vi "בדיקת מתח תפיסה של סליל פיקוד ללא עומס 5.vi"(8 "error":errorcluster, 10 "lines":tag="PXI1Slot8/port0/line1", 11 "Path for Log":path) -> (0 "error out":errorcluster, 1 "מצב ממסר פתוח/סגור":bool, 2 "מתח סגירת הממסר":dbl format="%.4f", 3 "מתח מוצא מהספק":dbl format="%.4f", 5 "resultUserPrompt":bool)   [LabVIEW 2015]
uses:
  <vilib>/DAQmx/write.llb/DAQmx Write (Digital Bool 1Line 1Point).vi
  <vilib>/DAQmx/create/channels.llb/DAQmx Create Channel (DO-Digital Output).vi
  <vilib>/DAQmx/miscellaneous.llb/DAQmx Fill In Error Info.vi
panel:
  out "progress":dbl(slide) scale=0.0..36.0
  out "error IO DMM":errorcluster
  in  "Stop Button":bool
  # "Right-Click to\nexplain error"
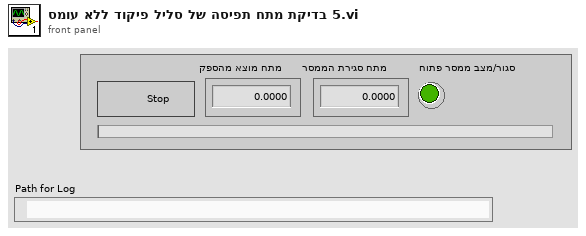
[diagram p1: front panel]
types:
  T1 = enum32{"Invalid", "Standard", "Closed", "Hidden", "Minimized", "Maximized"}
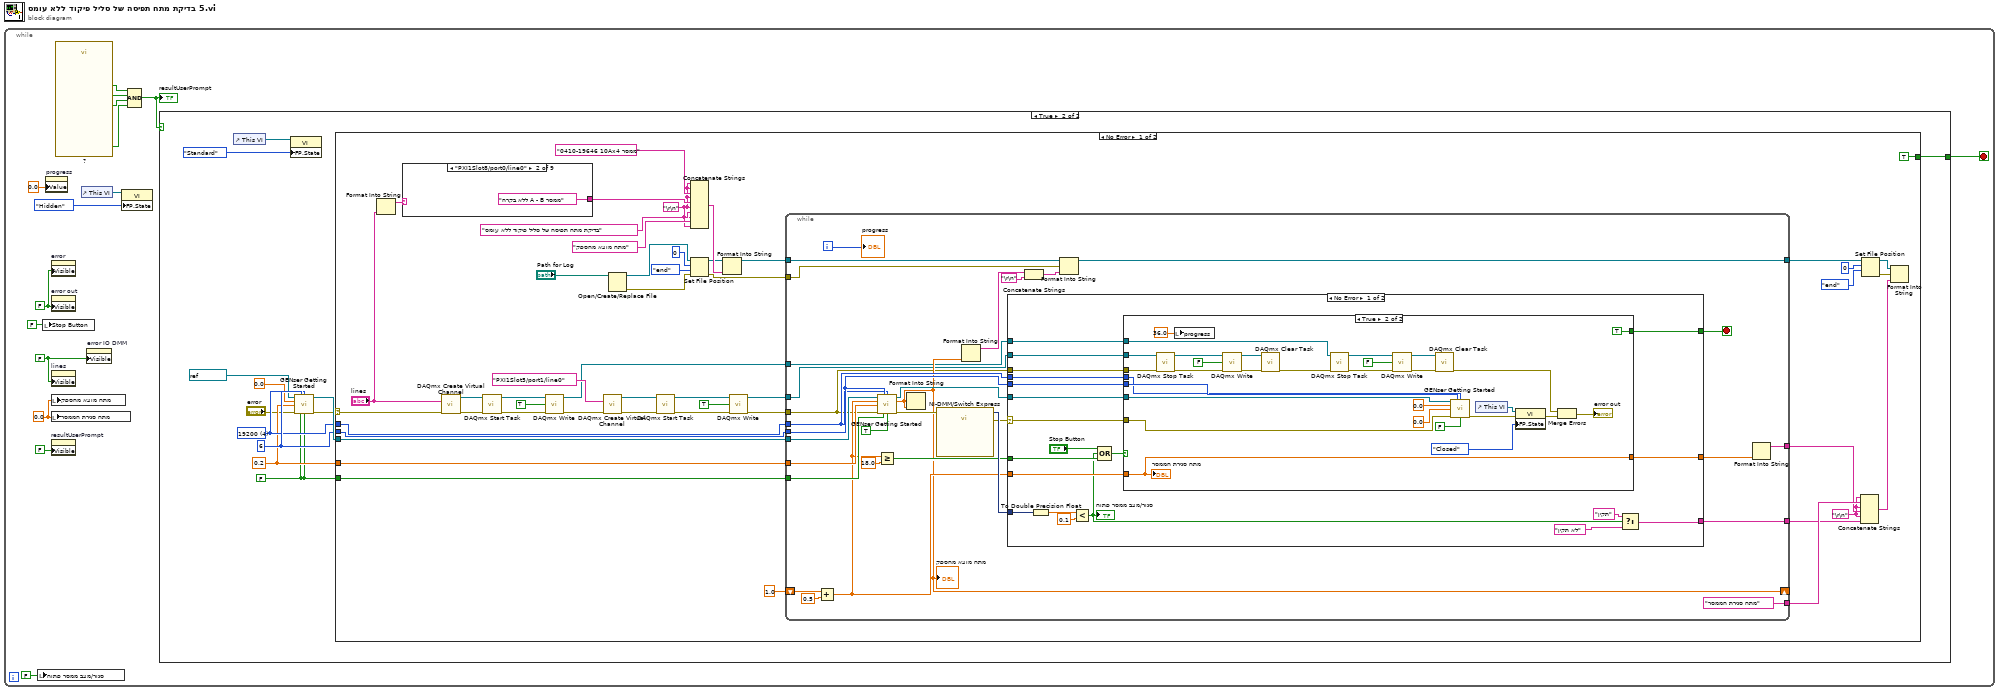
[diagram p0: block diagram]
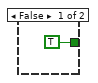
[diagram p2: hidden frame]
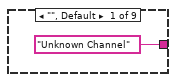
[diagram p3: hidden frame]
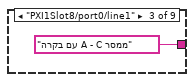
[diagram p4: hidden frame]
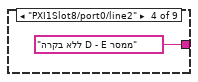
[diagram p5: hidden frame]
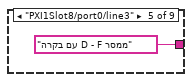
[diagram p6: hidden frame]
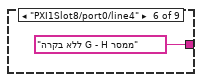
[diagram p7: hidden frame]
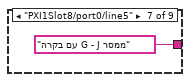
[diagram p8: hidden frame]
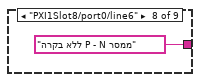
[diagram p9: hidden frame]
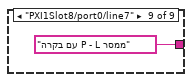
[diagram p10: hidden frame]
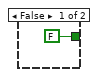
[diagram p11: hidden frame]
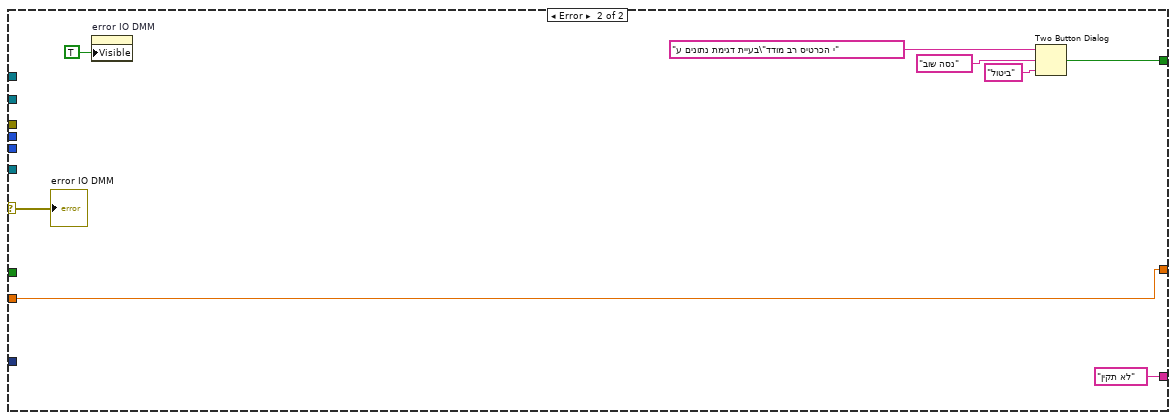
[diagram p12: hidden frame]
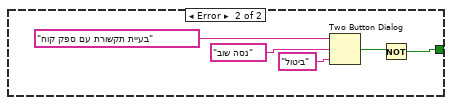
[diagram p13: hidden frame]
diagram:
  n1 = while {
    stop <- w1 stop-if-true
    w4 = FALSE ("Visible")
    w9 = 0.0 ("signals out")
    w2 = FALSE ("Visible")
    n2 = local write "מצב ממסר פתוח/סגור"(FALSE ("מגע סגור")) -> ()
    n3 = local write "Stop Button"(FALSE ("Reset (T)")) -> ()
    n4 = property on="progress" class="Slide (strict)"("Value"=0.0 ("progress")) -> ()  [unwired: 2 in, 2 out]
    n5 = property on="error" class="Clust (strict)"("Visible"=w4) -> ()  [unwired: 2 in, 2 out]
    n6 = property on="error out" class="Clust (strict)"("Visible"=w4) -> ()  [unwired: 2 in, 2 out]
    n7 = property on="lines" class="DAQmxName"("Visible"=w2) -> ()  [unwired: 2 in, 2 out]
    n8 = local write "מתח מוצא מהספק"(w9) -> ()
    n9 = local write "מתח סגירת הממסר"(w9) -> ()
    n10 = property on="resultUserPrompt" class="Bool (strict)"("Visible"=FALSE) -> ()  [unwired: 2 in, 2 out]
    n11 = call "?"() -> ("הדקי הרב מודד"=w7:bool, "M מגע שלילי"=w13:bool, "K מגע חיובי"=w14:bool, "OK"=w8:bool)  [unwired: 15 in, 1 out]
    n12 = control-ref of="This VI"() -> (w6:refnum<vi>)
    n13 = property on="error IO DMM" class="Clust (strict)"("Visible"=w2) -> ()  [unwired: 2 in, 2 out]
    n14 = property class="VI"(reference=w6, "FP.State"=T1."Hidden" ("Front Panel Window:State")) -> ()  [unwired: 1 in, 2 out]
    n15 = Compound Arithmetic op=AND(w8, w14, w13, w7) -> (w15:bool)
    "resultUserPrompt" <- w15
    n16 = case shown="True" w15 {
      tunnel: [TRUE ("T button?") w22] -> w1
      frame False {
      }
      frame True {
        w21 = FALSE ("Output On (T)")
        w26 = u16 4 items=["1200", "2400", "4800", "9600", "19200"] ("BAUD")
        w27 = i16 6 ("GEN Addr")
        w23 = 0.2 ("Current Limit")
        n17 = control-ref of="This VI"() -> (w19:refnum<vi>)
        n18 = property class="VI"(reference=w19, "FP.State"=T1."Standard" ("Front Panel Window:State")) -> ()  [unwired: 1 in, 2 out]
        n19 = call "GENser Getting Started.vi"("VISA"=refnum<visa-resource-name> "COM6", "GEN Addr"=w27, "BAUD"=w26, "Voltage Limit"=0.0, "Current Limit"=w23, "error"="error", "Reset (T)"=w21, "Output On (T)"=w21) -> ("VISA out"=w28:refnum<visa-resource-name>, "error out"=w18:errorcluster)  [unwired: 4 in, 2 out]
        n20 = case shown="No Error" w18 {
          selector: w18 -> [w45 _]
          tunnel: w28 -> [w77 _]
          tunnel: w27 -> [w76 _]
          tunnel: w26 -> [w75 _]
          tunnel: w21 -> [w74 _]
          tunnel: w23 -> [w73 _]
          tunnel: [TRUE w177] -> w22
          frame No Error {
            w29 = "\r\n"
            w67 = "\r\n"
            n21 = Format Into String("lines") -> (resulting string=w33:string)  [unwired: 3 in, 1 out]
            n22 = case shown="\"PXI1Slot8/port0/line0\"" w33 {
              tunnel: ["Unknown Channel" "ללא בקרה A - B ממסר" "עם בקרה A - C ממסר" "ללא בקרה D - E ממסר" "עם בקרה D - F ממסר" "ללא בקרה G - H ממסר" "עם בקרה G - J ממסר" "ללא בקרה P - N ממסר" "עם בקרה P - L ממסר"] -> w31
              frame "", Default {
              }
              frame "PXI1Slot8/port0/line0" {
              }
              frame "PXI1Slot8/port0/line1" {
              }
              frame "PXI1Slot8/port0/line2" {
              }
              frame "PXI1Slot8/port0/line3" {
              }
              frame "PXI1Slot8/port0/line4" {
              }
              frame "PXI1Slot8/port0/line5" {
              }
              frame "PXI1Slot8/port0/line6" {
              }
              frame "PXI1Slot8/port0/line7" {
              }
            }
            n23 = call-poly <vilib>:"DAQmx Create Virtual Channel.vi"("lines"="lines", "error in"=w45) -> ("task out"=w50:refnum<k21>, "error out"=w49:errorcluster)  [unwired: 12 in]
            n24 = call <vilib>:"DAQmx Start Task.vi"("task/channels in"=w50, "error in"=w49) -> ("task out"=w47:refnum<k21>, "error out"=w48:errorcluster)  [unwired: 12 in]
            n25 = call-poly <vilib>:"DAQmx Write.vi"("task/channels in"=w47, "data"=TRUE, "error in"=w48) -> ("task out"=w34:refnum<k21>, "error out"=w44:errorcluster)  [unwired: 10 in, 1 out]
            n26 = call-poly <vilib>:"DAQmx Create Virtual Channel.vi"("lines"=tag "PXI1Slot5/port1/line0", "error in"=w44) -> ("task out"=w57:refnum<k21>, "error out"=w58:errorcluster)  [unwired: 12 in]
            n27 = Open/Create/Replace File(file path (use dialog)="Path for Log") -> (refnum out=w41:refnum<file>, error out=w40:errorcluster)  [unwired: 5 in, 1 out]
            n28 = call <vilib>:"DAQmx Start Task.vi"("task/channels in"=w57, "error in"=w58) -> ("task out"=w54:refnum<k21>, "error out"=w53:errorcluster)  [unwired: 12 in]
            n29 = Concatenate Strings(w29, w29, "0410-19646 10Ax4 ממסר", w29, w31, w29, "בדיקת מתח תפיסה של סליל פיקוד ללא עומס", w29, "מתח מוצא מהספק", w29) -> (w39:string)
            n30 = Set File Position(offset (in bytes) (0)=i64 0, refnum=w41, from (0:start)=enum16{"start", "end", "current"}."end", error in=w40) -> (refnum out=w36:refnum<file>, error out=w60:errorcluster)
            n31 = Format Into String(initial string=w36, w39) -> (resulting string=w59:refnum<file>)  [unwired: 2 in, 1 out]
            n32 = call-poly <vilib>:"DAQmx Write.vi"("task/channels in"=w54, "data"=TRUE, "error in"=w53) -> ("task out"=w52:refnum<k21>, "error out"=w51:errorcluster)  [unwired: 10 in, 1 out]
            n33 = while {
              tunnel: w77 -> [w107]
              tunnel: w76 -> [w109]
              tunnel: w75 -> [w108]
              tunnel: w74 -> [w117]
              tunnel: w73 -> [w115]
              shift-right: [w99] -> _
              shift-left: 1.0 ("y") -> [w113]
              tunnel: ["מתח סגירת הממסר"] -> w70
              tunnel: [w97] -> w69
              tunnel: [w96] -> w68
              tunnel: [w93] -> w66
              tunnel: w59 -> [w92]
              tunnel: w60 -> [w91]
              tunnel: w52 -> [w89]
              tunnel: w51 -> [w88]
              tunnel: w34 -> [w87]
              i -> [w100]
              stop <- w110 stop-if-true
              n34 = Add(x=w113, y=0.5) -> (x+y=w101:dbl)
              n35 = call "GENser Getting Started.vi"("VISA"=w107, "GEN Addr"=w109, "BAUD"=w108, "Voltage Limit"=w101, "Current Limit"=w115, "error"=w88, "Reset (T)"=w117, "Output On (T)"=TRUE) -> ("VISA out"=w106:refnum<visa-resource-name>, "Output Voltage"=w99:dbl, "error out"=w112:errorcluster)  [unwired: 4 in, 1 out]
              "מתח מוצא מהספק" <- w99
              n36 = Greater Or Equal?(x=w101, y=18.0) -> (x >= y?=w104:bool)
              n37 = Format Into String(w99) -> ()  [unwired: 3 in, 2 out]
              n38 = call "NI-DMM/Switch Express"("error in"=w112) -> ("signals out"=w111:dynamicdata, "error out"=w103:errorcluster)  [unwired: 16 in, 1 out]
              n39 = Format Into String(w99) -> (resulting string=w94:string)  [unwired: 3 in, 1 out]
              n40 = case shown="No Error" w103 {
                selector: w103 -> [w129 w176]
                tunnel: w111 -> [w137 _]
                tunnel: [w126 w172] -> w110
                tunnel: w109 -> [w134 _]
                tunnel: w108 -> [w133 _]
                tunnel: w106 -> [w132 _]
                tunnel: w104 -> [w131 _]
                tunnel: w101 -> [w130 w170]
                tunnel: [w125 w170] -> w102
                tunnel: [w122 "לא תקין"] -> w96
                tunnel: w89 -> [w120 _]
                tunnel: w88 -> [w119 _]
                tunnel: w87 -> [w118 _]
                frame No Error {
                  n41 = To Double Precision Float(number=w137) -> (double precision float=w128:dbl)
                  n42 = Less?(x=w128, y=0.1) -> (x < y?=w121:bool)
                  "מצב ממסר פתוח/סגור" <- w121
                  n43 = Compound Arithmetic op=OR("Stop Button", w121, w131) -> (w136:bool)
                  n44 = case shown="True" w136 {
                    tunnel: [FALSE TRUE] -> w126
                    tunnel: w134 -> [_ w168]
                    tunnel: w133 -> [_ w167]
                    tunnel: w132 -> [_ w166]
                    tunnel: w129 -> [_ w163]
                    tunnel: w130 -> [_ w158]
                    tunnel: [_ w158] -> w125
                    tunnel: w120 -> [_ w149]
                    tunnel: w119 -> [_ w148]
                    tunnel: w118 -> [_ w139]
                    frame False {
                    }
                    frame True {
                      n45 = call <vilib>:"DAQmx Stop Task.vi"("task/channels in"=w149, "error in"=w148) -> ("task out"=w156:refnum<k21>, "error out"=w154:errorcluster)  [unwired: 12 in]
                      n46 = local write "progress"(36.0 ("progress")) -> ()
                      n47 = call-poly <vilib>:"DAQmx Write.vi"("task/channels in"=w156, "data"=FALSE, "error in"=w154) -> ("task out"=w153:refnum<k21>, "error out"=w152:errorcluster)  [unwired: 10 in, 1 out]
                      n48 = call <vilib>:"DAQmx Clear Task.vi"("task in"=w153, "error in"=w152) -> ("error out"=w141:errorcluster)  [unwired: 13 in]
                      n49 = call <vilib>:"DAQmx Stop Task.vi"("task/channels in"=w139, "error in"=w141) -> ("task out"=w142:refnum<k21>, "error out"=w144:errorcluster)  [unwired: 12 in]
                      n50 = call-poly <vilib>:"DAQmx Write.vi"("task/channels in"=w142, "data"=FALSE, "error in"=w144) -> ("task out"=w145:refnum<k21>, "error out"=w146:errorcluster)  [unwired: 10 in, 1 out]
                      n51 = call <vilib>:"DAQmx Clear Task.vi"("task in"=w145, "error in"=w146) -> ("error out"=w140:errorcluster)  [unwired: 13 in]
                      n52 = call "GENser Getting Started.vi"("VISA"=w166, "GEN Addr"=w168, "BAUD"=w167, "Voltage Limit"=0.0, "Current Limit"=0.0, "error"=w163, "Output On (T)"=FALSE) -> ("error out"=w147:errorcluster)  [unwired: 5 in, 3 out]
                      n53 = control-ref of="This VI"() -> (w160:refnum<vi>)
                      n54 = property class="VI"(reference=w160, error in=w147, "FP.State"=T1."Closed" ("Front Panel Window:State")) -> (error out=w150:errorcluster)  [unwired: 1 out]
                      n55 = Merge Errors(w140, w150) -> (→"error out":errorcluster)
                      "מתח סגירת הממסר" <- w158
                    }
                  }
                  n56 = Select(t="תקין", s=w121, f="לא תקין") -> (s? t:f=w122:string)
                }
                frame Error {
                  n57 = property on="error IO DMM" class="Clust (strict)"("Visible"=TRUE) -> ()  [unwired: 2 in, 2 out]
                  n58 = Two Button Dialog(message="בעיית דגימת נתונים ע\"י הכרטיס רב מודד", 1:"ביטול" ("F button name (\"Cancel\")"), 2:"נסה שוב" ("T button name (\"OK\")")) -> (T button?=w172:bool)
                  "error IO DMM" <- w176
                }
              }
              n59 = Concatenate Strings(w94, "\r\n") -> (w90:string)
              n60 = Format Into String(initial string=w92, error in=w91, w90) -> (resulting string=w93:refnum<file>)  [unwired: 1 in, 1 out]
              n61 = Format Into String(w102) -> (resulting string=w97:string)  [unwired: 3 in, 1 out]
              "progress" <- w100
            }
            n62 = Concatenate Strings(w67, w70, w67, w69, w67, w68) -> (w61:string)
            n63 = Set File Position(offset (in bytes) (0)=i64 0, refnum=w66, from (0:start)=enum16{"start", "end", "current"}."end") -> (refnum out=w63:refnum<file>, error out=w62:errorcluster)  [unwired: 1 in]
            n64 = Format Into String(initial string=w63, error in=w62, w61) -> ()  [unwired: 1 in, 2 out]
          }
          frame Error {
            n65 = Two Button Dialog(message="בעיית תקשורת עם ספק קוח", 1:"ביטול" ("F button name (\"Cancel\")"), 2:"נסה שוב" ("T button name (\"OK\")")) -> (T button?=w178:bool)
            n66 = Not(x=w178) -> (.not. x?=w177:bool)
          }
        }
      }
    }
  }
